vi "TEST PFIO Terminal.vi"   [LabVIEW 2017]
uses:
  <vilib>/DAQmx/configure/timing.llb/DAQmx Timing (Sample Clock).vi
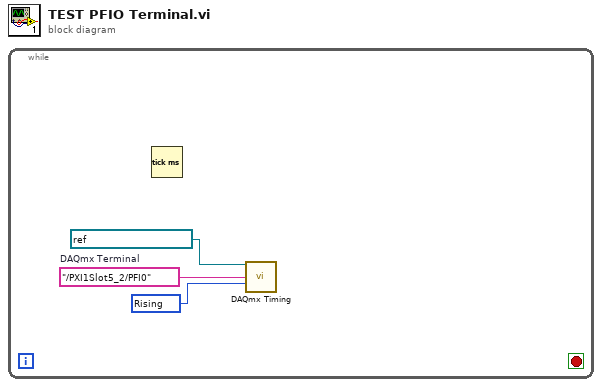
[diagram p0: block diagram]
diagram:
  n1 = while {
    stop <- _ stop-if-true
    w2 = 10280 items=["Rising"=10280, "Falling"=10171] ("active edge")
    w3 = tag "/PXI1Slot5_2/PFI0"  # DAQmx Terminal
    n2 = Tick Count (ms)() -> ()  [unwired: 1 out]
    n3 = call-poly <vilib>:"DAQmx Timing.vi"("task/channels in"=refnum<k21> "Slot 5 - AI Current", "source"=w3, "active edge"=w2) -> ()  [unwired: 11 in, 2 out]
  }
